vi "StdFileName_LS1.vi"(7 "chemin de base":path, 8 "error in (no error)":errorcluster, 9 "Date":string, 10 "Scan":i64, 11 "Session":i32) -> (0 "error out":errorcluster, 2 "chemin Data":path, 3 "chemin Headers":path, 4 "Data Exist":bool, 5 "Hdr Exist":bool)   [LabVIEW 2010]
doc: "Ce VI sauvegarde les données d'acquisition pour en garder une copie de sécurité qui peut être rappeller en cas de panne."
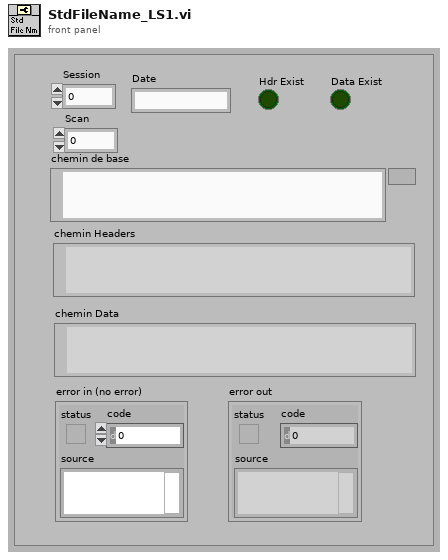
[diagram p1: front panel]
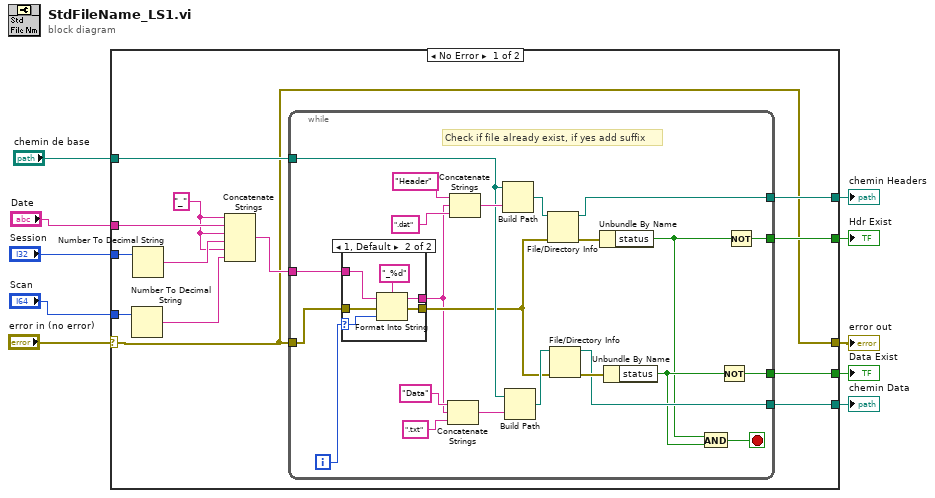
[diagram p0: block diagram]
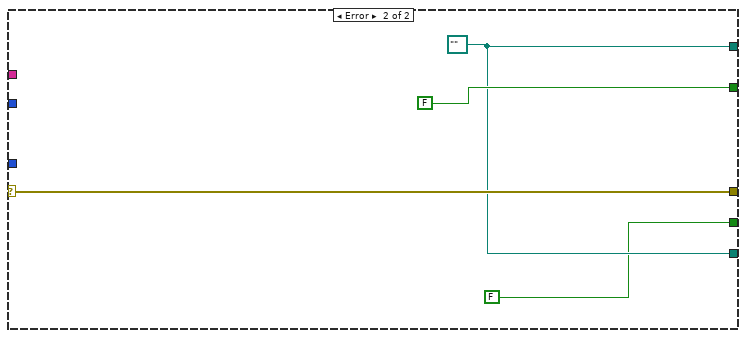
[diagram p3: hidden frame]
diagram:
  n1 = case shown="No Error" "error in (no error)" {
    selector: "error in (no error)" -> [w11 w57]
    tunnel: [w11 w57] -> w9
    tunnel: "Session" -> [w23 _]
    tunnel: "Date" -> [w22 _]
    tunnel: [w14 FALSE] -> w6
    tunnel: [w12 w55] -> w5
    tunnel: [w20 w55] -> w4
    tunnel: [w19 FALSE] -> w3
    tunnel: "Scan" -> [w18 _]
    tunnel: "chemin de base" -> [w15 _]
    frame No Error {
      w16 = "_" ("name or relative path")
      n2 = Number To Decimal String(number=w18) -> (decimal integer string=w17:string)  [unwired: 1 in]
      n3 = Number To Decimal String(number=w23) -> (decimal integer string=w21:string)  [unwired: 1 in]
      n4 = Concatenate Strings(w16, w22, w16, w21, w16, w17) -> (w13:string)
      n5 = while {
        tunnel: [w39] -> w20
        tunnel: [w33] -> w19
        tunnel: w15 -> [w36]
        tunnel: [w32] -> w14
        tunnel: w13 -> [w30]
        tunnel: [w34] -> w12
        tunnel: w11 -> [w29]
        i -> [w24]
        stop <- w31 stop-if-true
        # "Check if file already exist, if yes add suffix"
        n6 = case shown="1, Default" w24 {
          selector: w24 -> [_ w48]
          tunnel: w30 -> [w47 w49]
          tunnel: w29 -> [w46 w52]
          tunnel: [w46 w51] -> w28
          tunnel: [w47 w50] -> w27
          frame 0 {
          }
          frame 1, Default {
            n7 = Format Into String(format string="_%d" ("chaîne de format"), initial string=w49, error in=w52, w48) -> (resulting string=w50:string, error out=w51:errorcluster)
          }
        }
        n8 = Concatenate Strings("Data" ("chaîne"), w27, ".txt" ("name or relative path")) -> (w43:string)
        n9 = Concatenate Strings("Header" ("chaîne"), w27, ".dat" ("name or relative path")) -> (w44:string)
        n10 = Build Path(base path=w36, name or relative path=w44) -> (appended path=w35:path)
        n11 = Build Path(base path=w36, name or relative path=w43) -> (appended path=w39:path)
        n12 = File/Directory Info(path=w35, error in=w28) -> (path out=w34:path, error out=w45:errorcluster)  [unwired: 5 out]
        n13 = File/Directory Info(path=w39, error in=w28) -> (error out=w40:errorcluster)  [unwired: 6 out]
        n14 = Unbundle By Name(w45) -> ("status"=w25:bool)
        n15 = Unbundle By Name(w40) -> ("status"=w26:bool)
        n16 = And(x=w25, y=w26) -> (x .and. y?=w31:bool)
        n17 = Not(x=w26) -> (.not. x?=w33:bool)
        n18 = Not(x=w25) -> (.not. x?=w32:bool)
      }
    }
    frame Error {
      w55 = path "" ("appended path")
    }
  }
  "error out" <- w9
  "Hdr Exist" <- w6
  "chemin Headers" <- w5
  "chemin Data" <- w4
  "Data Exist" <- w3
